vi "_main__.vi"() -> ()   [LabVIEW 2015]
doc: "PKT-8 based Magnitometer"
uses:
  <vilib>/NI/Modbus Library/API/Master/Modbus Master.lvclass
  Load and Save Controls_LV2009.llb/RWC_Actions.ctl
  <vilib>/Utility/error.llb/DialogType.ctl
panel:
  out "ch8_z":dbl format="%.1f"
  out "ch7_z":dbl format="%.1f"
  out "ch6_z":dbl format="%.1f"
  out "ch5_z":dbl format="%.1f"
  out "ch4_z":dbl format="%.1f"
  out "ch3_z":dbl format="%.1f"
  out "ch2_z":dbl format="%.1f"
  out "ch1_z":dbl format="%.1f"
  out "new point":bool=TRUE
  out "статус":bool
  in  "счетчик":u16
  in  "Tab Control":enum32{"Изм.", "Н 1", "Н 2"}(tab)
  in  "show graph B":bool
  in  "show graph U":bool
  out "U8":dbl format="%.1f"
  out "U7":dbl format="%.1f"
  out "U6":dbl format="%.1f"
  out "U5":dbl format="%.1f"
  out "U4":dbl format="%.1f"
  out "U3":dbl format="%.1f"
  out "U2":dbl format="%.1f"
  out "U1":dbl format="%.1f"
  out "8":dbl format="%.2f"
  out "7":dbl format="%.2f"
  out "6":dbl format="%.2f"
  out "5":dbl format="%.2f"
  out "4":dbl format="%.2f"
  out "3":dbl format="%.2f"
  out "2":dbl format="%.2f"
  out "1":dbl format="%.3f"
  in  "Режим работы графика":enum32{"Самописец", "Ручное упр."}(radio)
  in  "Add point":bool
  in  "buf en":bool=TRUE caption="1_ch_abs 2"
  in  "buffer":u16=20 min=1 max=128
  in  "SPS":enum16{"2,5 SPS", "5 SPS", "10 SPS"}(ring)=enum."5 SPS"
  in  "ID":u8=102
  in  "Порт":u16
  in  "IP":string
  in  "Пароль":string
  out "refnum out":refnum<file>
  in  "stop":bool
  in  "range":T1(ring)=enum."± 312.5 мВ"
  in  "Set_zero_8":bool
  in  "Set_zero_7":bool
  in  "Set_zero_6":bool
  in  "Set_zero_5":bool
  in  "Set_zero_4":bool
  in  "Set_zero_3":bool
  in  "Set_zero_2":bool
  in  "Set_zero_1":bool
  in  "канал 1":dbl=76.0 format="%#_4g"
  in  "канал 2":dbl=76.0 format="%#_4g"
  in  "канал 3":dbl=76.0 format="%#_4g"
  in  "канал 4":dbl=76.0 format="%#_4g"
  in  "канал 5":dbl=76.0 format="%#_4g"
  in  "канал 6":dbl=76.0 format="%#_4g"
  in  "канал 7":dbl=76.0 format="%#_4g"
  in  "канал 8":dbl=76.0 format="%#_4g"
  in  "Сохранение в файл":bool=TRUE
  in  "интервал, сек.":u16=30 min=1 max=3600 step=1
  out "Path":string
  out "File header exist?":bool caption="Disconn"
  out "Соед.":refnum<class "Modbus Master.lvclass">
  # "№"
  # "B [ mT ]"
  # "U [ uV ]"
  # "Настройки АЦП"
  # "Буфер. усреднения"
  # "Скорость измерений"
  # "SPS = Samples Per Sec."
  # "Диапазон"
  # "Входной буфер АЦП"
  # "Настройки соединения"
  # "Пароль"
  # "Коэффициенты, uV/mT"
  # "Установка нуля"
  # "Настройки сохранения"
types:
  T1 = enum16{"", "± 2.5 В", "± 1.25 В", "± 0.625 В", "± 312.5 мВ", "± 156.25 мВ", "± 78.125 мВ"}
  T2 = typedef "DialogType.ctl" = u16
  T3 = typedef "RWC_Actions.ctl" = enum16{"Read", "Write", "Read and Create"}
  T4 = enum8{"Enabled", "Disabled", "Disabled and Grayed Out"}
  T5 = cluster{"U1":dbl, "U2":dbl, "U3":dbl, "U4":dbl, "U5":dbl, "U6":dbl, "U7":dbl, "U8":dbl}
  T6 = cluster{"1":dbl, "2":dbl, "3":dbl, "4":dbl, "5":dbl, "6":dbl, "7":dbl, "8":dbl}
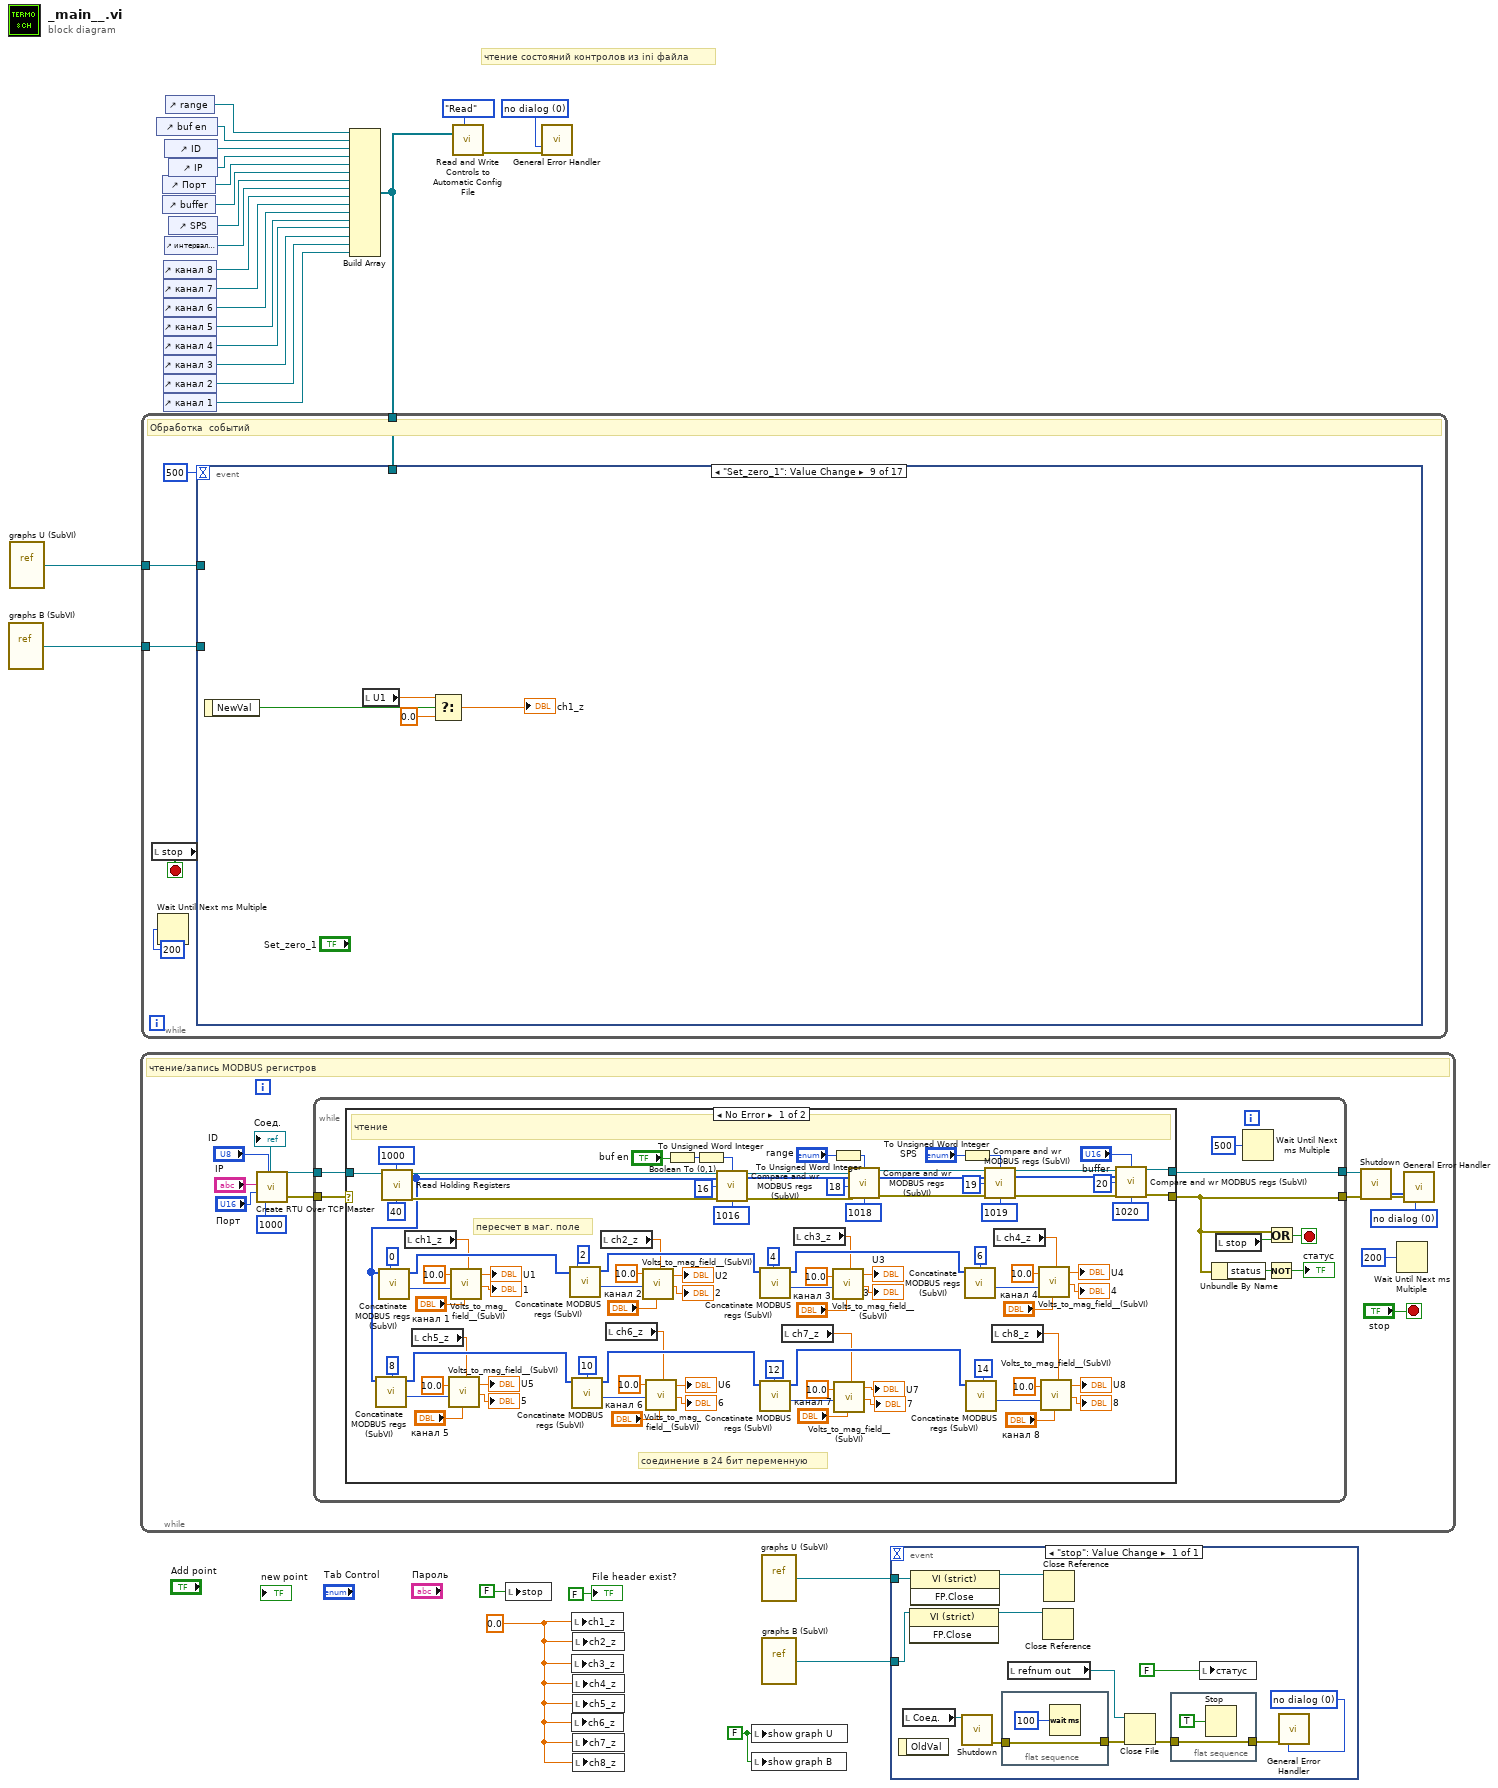
[diagram p0: block diagram]
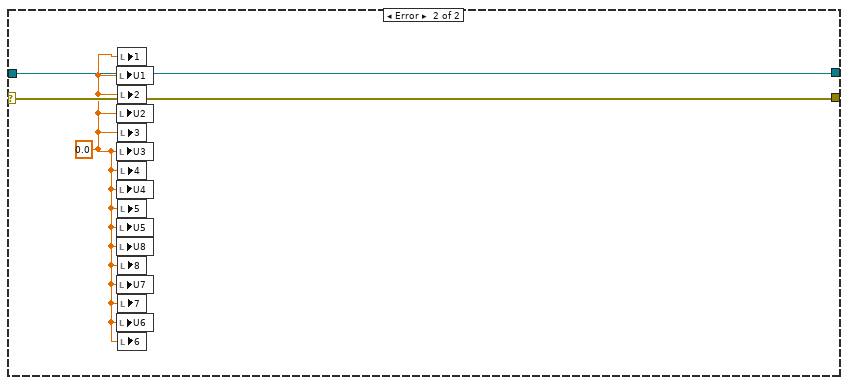
[diagram p2: hidden frame]
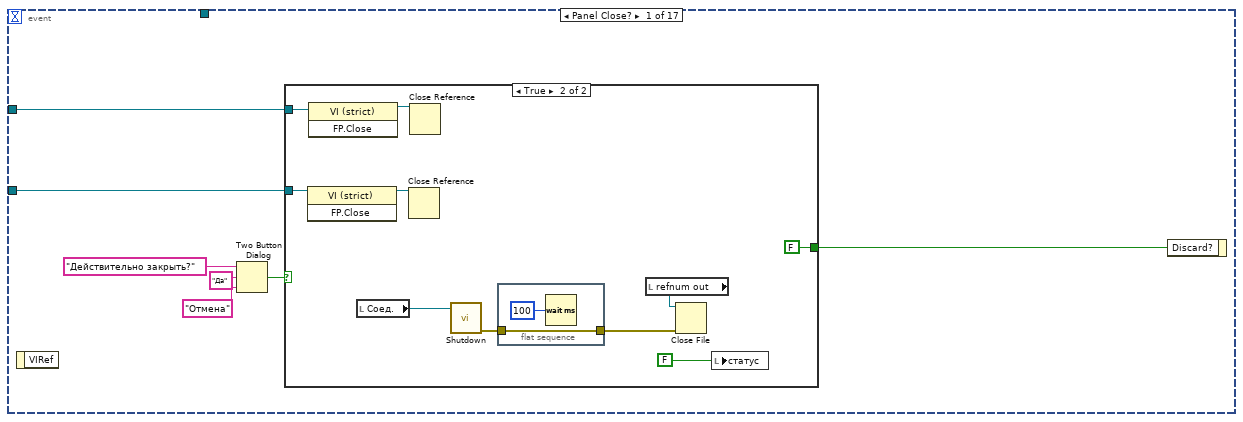
[diagram p3: hidden frame]
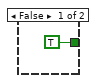
[diagram p4: hidden frame]
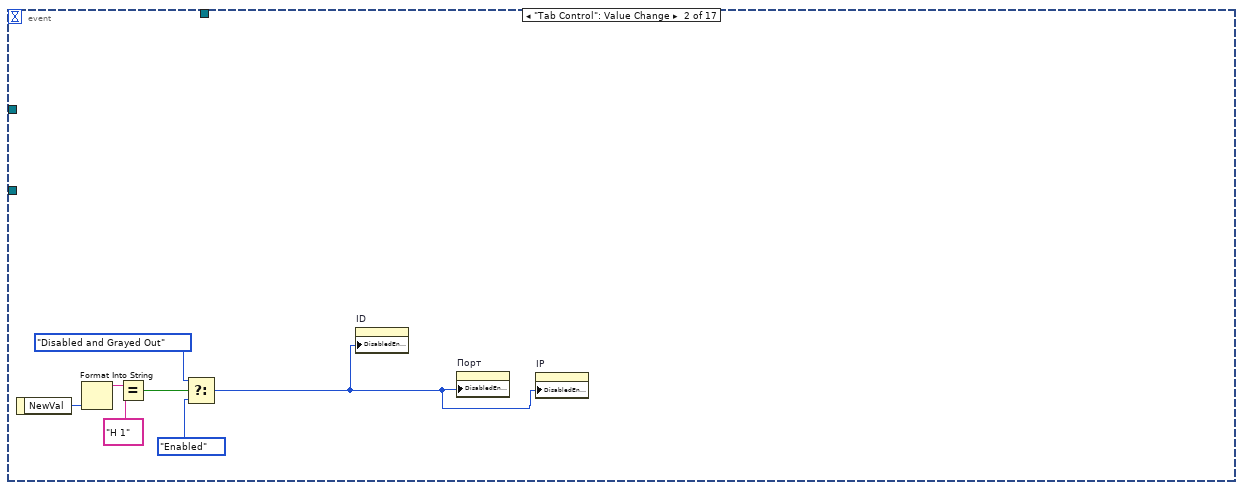
[diagram p5: hidden frame]
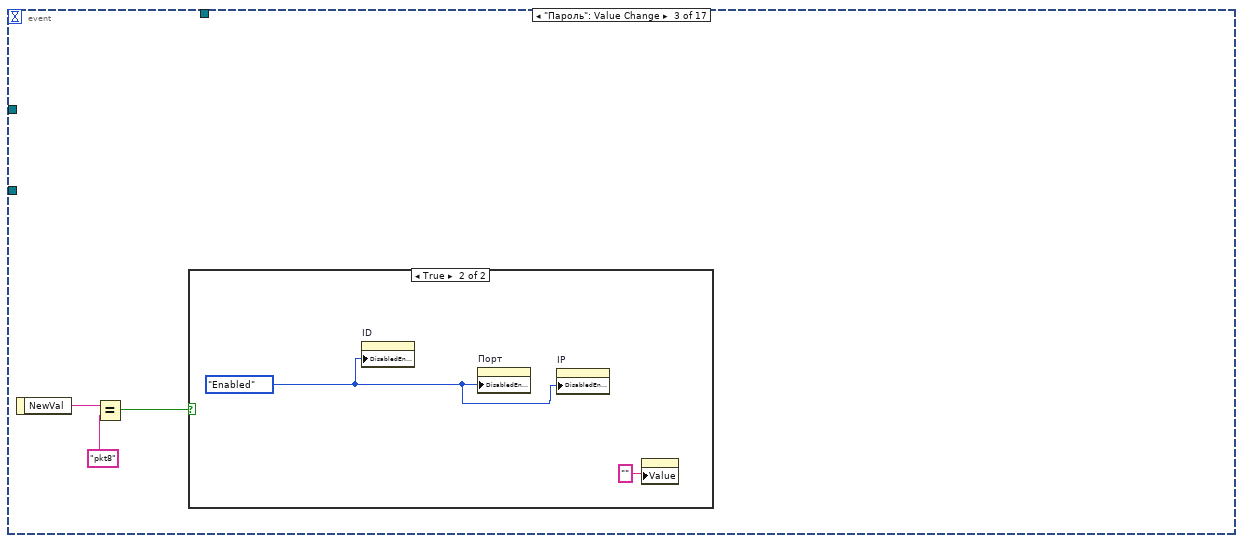
[diagram p6: hidden frame]
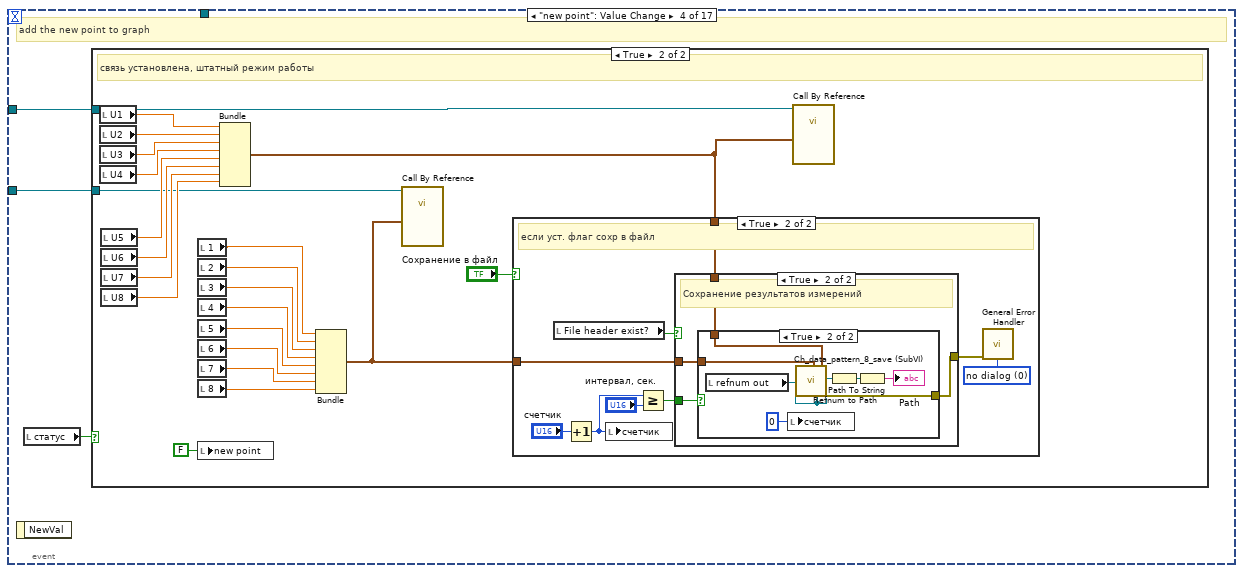
[diagram p8: hidden frame]
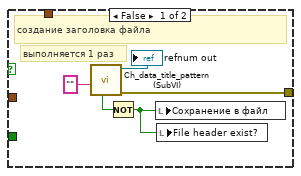
[diagram p11: hidden frame]
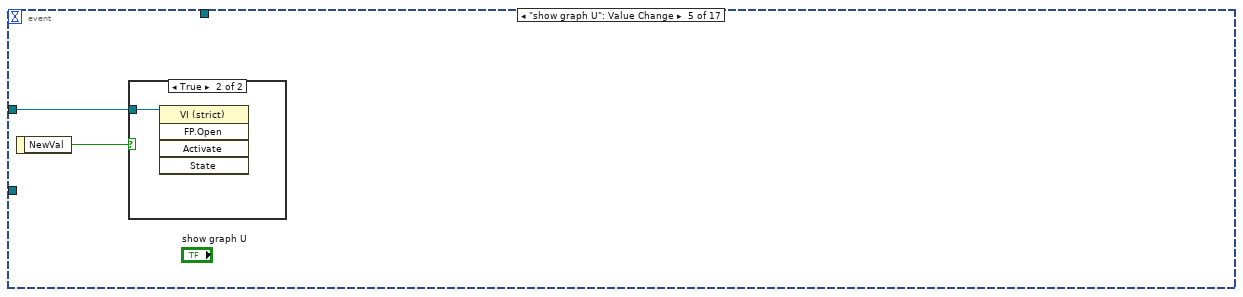
[diagram p13: hidden frame]
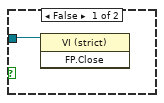
[diagram p14: hidden frame]
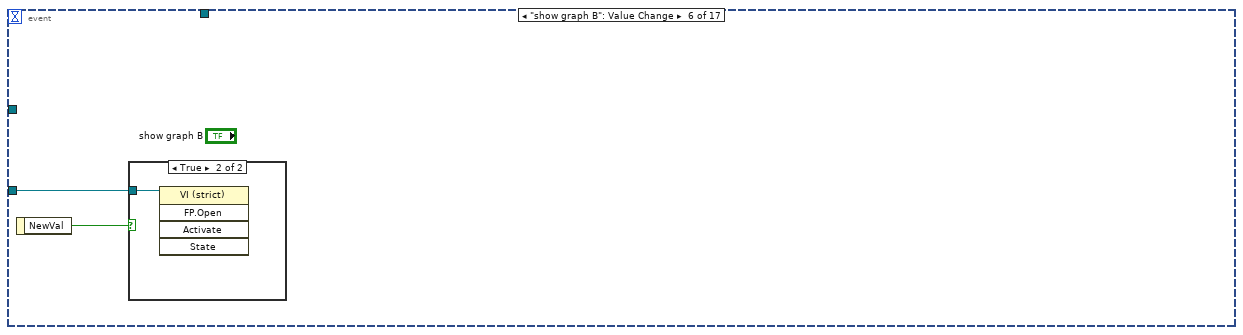
[diagram p15: hidden frame]
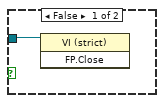
[diagram p16: hidden frame]
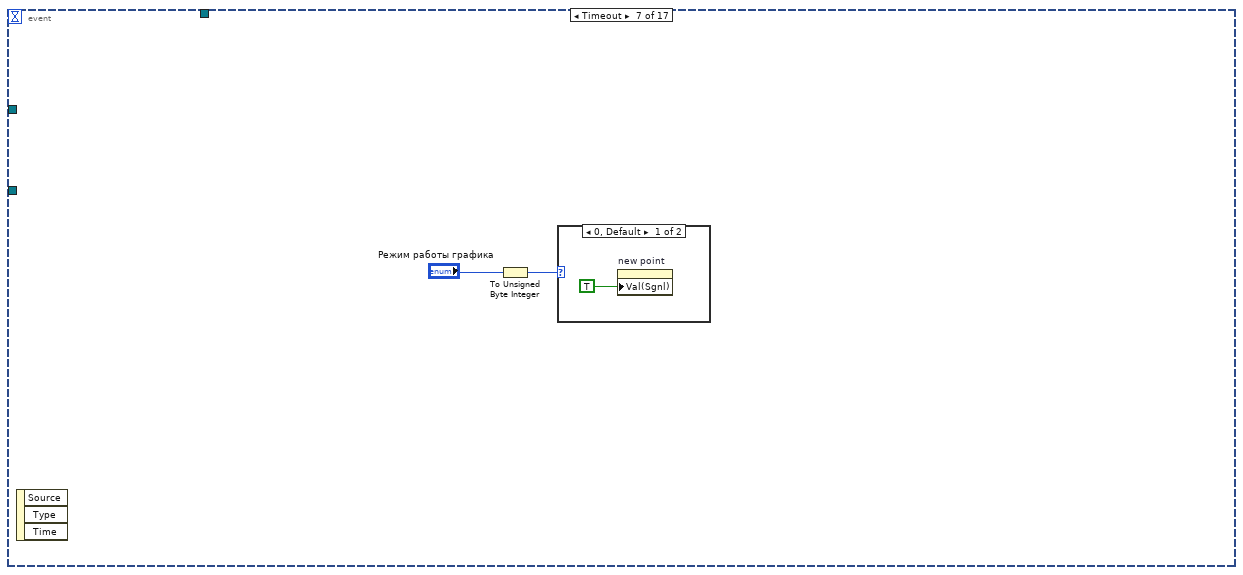
[diagram p17: hidden frame]
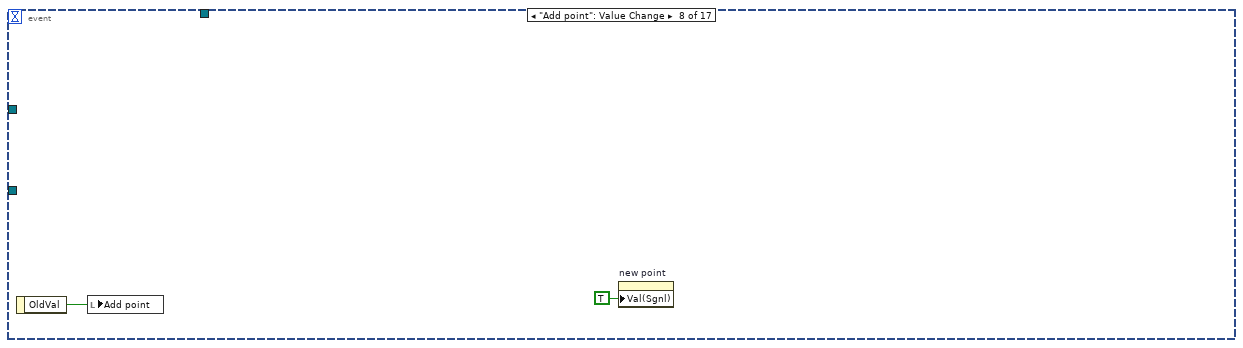
[diagram p19: hidden frame]
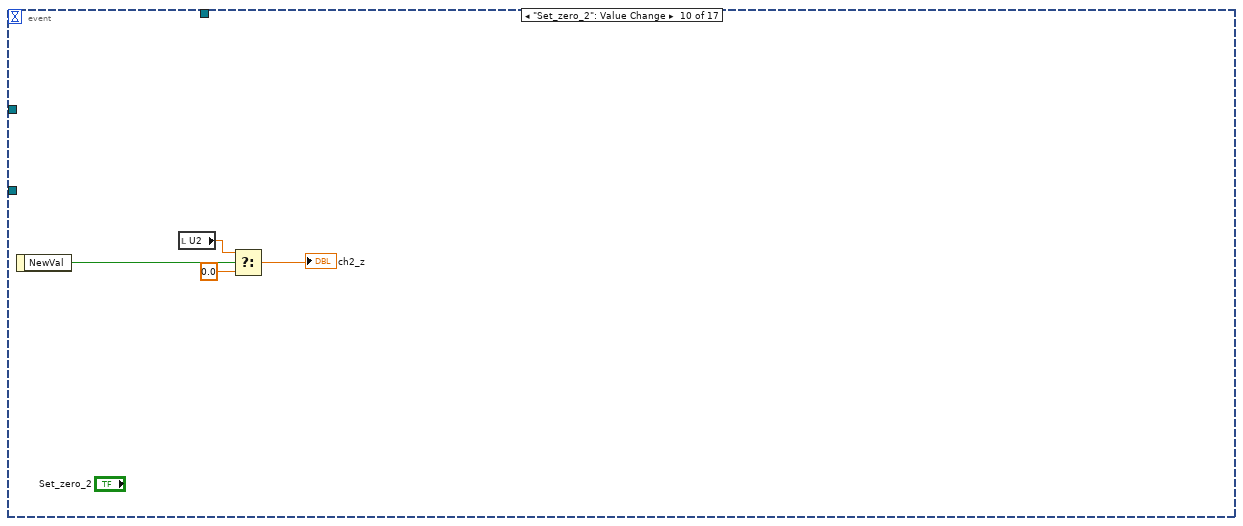
[diagram p20: hidden frame]
diagram:
  w2 = 0.0 ("U1")
  w4 = FALSE ("show graph U")
  w20 = T2 0 items=["no dialog", "OK message", "continue or stop message", "OK message + warnings", "continue/stop + warnings"] ("type of dialog (OK msg:1)")
  # "чтение состояний контролов из ini файла"
  n1 = vi-ref "graphs B (SubVI).vi"() -> (w5:refnum<vi>)
  n2 = vi-ref "graphs U (SubVI).vi"() -> (w8:refnum<vi>)
  n3 = while {
    stop <- "stop" stop-if-true
    w32 = T2 0 items=["no dialog", "OK message", "continue or stop message", "OK message + warnings", "continue/stop + warnings"] ("type of dialog (OK msg:1)")
    # "чтение/запись MODBUS регистров"
    n4 = call "Create RTU Over TCP Master.vi"("unit ID"="ID", "connect timeout ms"=1000, "port (502)"="Порт", "address"="IP") -> ("error out"=w36:errorcluster, "TCP master instance"=w37:refnum<class "Modbus Master.lvclass">)  [unwired: 6 in]
    "Соед." <- w37
    n5 = while {
      tunnel: w37 -> [w49]
      tunnel: w36 -> [w48]
      tunnel: [w42] -> w35
      tunnel: [w47] -> w34
      stop <- w45 stop-if-true
      n6 = case shown="No Error" w48 {
        selector: w48 -> [_ w146]
        tunnel: w49 -> [w142 w147]
        tunnel: [w99 w146] -> w42
        tunnel: [w100 w147] -> w47
        frame No Error {
          # "пересчет в маг. поле"
          # "соединение в 24 бит переменную"
          # "чтение"
          n7 = call-dynamic "Read Holding Registers.vi"("number of inputs"=u16 40, "starting address"=u16 1000, "Modbus master in"=w142) -> ("error out"=w101:errorcluster, "register values"=w58:u16[], "Modbus master out"=w102:refnum<class "Modbus Master.lvclass">)  [unwired: 6 in]
          n8 = call "Concatinate MODBUS regs (SubVI).vi"("LSB reg num"=u16 8, "registers array in"=w58) -> ("register data"=w124:i32, "registers array out"=w86:u16[])  [unwired: 8 in]
          n9 = call "Concatinate MODBUS regs (SubVI).vi"("LSB reg num"=u16 0, "registers array in"=w58) -> ("register data"=w129:i32, "registers array out"=w89:u16[])  [unwired: 8 in]
          n10 = local read "ch1_z"() -> (w57:dbl)
          n11 = local read "ch5_z"() -> (w53:dbl)
          n12 = call "Volts_to_mag_field__(SubVI).vi"("делитель"=10.0, "U"=w124, "k"="канал 5", "zero lvl"=w53) -> ("meas_voltage"=→"U5":dbl, "B"=→"5":dbl)  [unwired: 20 in, 2 out]
          n13 = call "Volts_to_mag_field__(SubVI).vi"("делитель"=10.0, "U"=w129, "k"="канал 1", "zero lvl"=w57) -> ("meas_voltage"=→"U1":dbl, "B"=→"1":dbl)  [unwired: 20 in, 2 out]
          n14 = call "Concatinate MODBUS regs (SubVI).vi"("LSB reg num"=u16 2, "registers array in"=w89) -> ("register data"=w128:i32, "registers array out"=w88:u16[])  [unwired: 8 in]
          n15 = call "Concatinate MODBUS regs (SubVI).vi"("LSB reg num"=u16 10, "registers array in"=w86) -> ("register data"=w123:i32, "registers array out"=w85:u16[])  [unwired: 8 in]
          n16 = local read "ch2_z"() -> (w56:dbl)
          n17 = local read "ch6_z"() -> (w52:dbl)
          n18 = call "Volts_to_mag_field__(SubVI).vi"("делитель"=10.0, "U"=w128, "k"="канал 2", "zero lvl"=w56) -> ("meas_voltage"=→"U2":dbl, "B"=→"2":dbl)  [unwired: 20 in, 2 out]
          n19 = call "Volts_to_mag_field__(SubVI).vi"("делитель"=10.0, "U"=w123, "k"="канал 6", "zero lvl"=w52) -> ("meas_voltage"=→"U6":dbl, "B"=→"6":dbl)  [unwired: 20 in, 2 out]
          n20 = Boolean To (0,1)(Boolean="buf en") -> (0, 1=w71:i16)
          n21 = To Unsigned Word Integer(number=w71) -> (unsigned 16bit integer=w70:u16)
          n22 = call "Compare and wr MODBUS regs (SubVI).vi"("Modbus Master in"=w102, "control"=w70, "modbus read arr in"=w58, "arr el. index"=16 ("arr element"), "error in (no error)"=w101, "reg address"=u16 1016 ("starting address")) -> ("Modbus Master out"=w81:refnum<class "Modbus Master.lvclass">, "modbus read arr  out"=w83:u16[], "error out"=w82:errorcluster)  [unwired: 7 in]
          n23 = call "Concatinate MODBUS regs (SubVI).vi"("LSB reg num"=u16 4, "registers array in"=w88) -> ("register data"=w127:i32, "registers array out"=w87:u16[])  [unwired: 8 in]
          n24 = call "Concatinate MODBUS regs (SubVI).vi"("LSB reg num"=u16 12, "registers array in"=w85) -> ("register data"=w122:i32, "registers array out"=w84:u16[])  [unwired: 8 in]
          n25 = local read "ch7_z"() -> (w51:dbl)
          n26 = local read "ch3_z"() -> (w55:dbl)
          n27 = To Unsigned Word Integer(number="range") -> (unsigned 16bit integer=w67:u16)
          n28 = call "Volts_to_mag_field__(SubVI).vi"("делитель"=10.0, "U"=w127, "k"="канал 3", "zero lvl"=w55) -> ("meas_voltage"=→"U3":dbl, "B"=→"3":dbl)  [unwired: 20 in, 2 out]
          n29 = call "Volts_to_mag_field__(SubVI).vi"("делитель"=10.0, "U"=w122, "k"="канал 7", "zero lvl"=w51) -> ("meas_voltage"=→"U7":dbl, "B"=→"7":dbl)  [unwired: 20 in, 2 out]
          n30 = call "Compare and wr MODBUS regs (SubVI).vi"("Modbus Master in"=w81, "control"=w67, "modbus read arr in"=w83, "arr el. index"=18 ("arr element"), "error in (no error)"=w82, "reg address"=u16 1018 ("starting address")) -> ("Modbus Master out"=w79:refnum<class "Modbus Master.lvclass">, "modbus read arr  out"=w78:u16[], "error out"=w80:errorcluster)  [unwired: 7 in]
          n31 = To Unsigned Word Integer(number="SPS") -> (unsigned 16bit integer=w63:u16)
          n32 = call "Concatinate MODBUS regs (SubVI).vi"("LSB reg num"=u16 6, "registers array in"=w87) -> ("register data"=w125:i32)  [unwired: 8 in, 1 out]
          n33 = call "Concatinate MODBUS regs (SubVI).vi"("LSB reg num"=u16 14, "registers array in"=w84) -> ("register data"=w121:i32)  [unwired: 8 in, 1 out]
          n34 = call "Compare and wr MODBUS regs (SubVI).vi"("Modbus Master in"=w79, "control"=w63, "modbus read arr in"=w78, "arr el. index"=19 ("arr element"), "error in (no error)"=w80, "reg address"=u16 1019 ("starting address")) -> ("Modbus Master out"=w76:refnum<class "Modbus Master.lvclass">, "modbus read arr  out"=w75:u16[], "error out"=w77:errorcluster)  [unwired: 7 in]
          n35 = local read "ch8_z"() -> (w50:dbl)
          n36 = local read "ch4_z"() -> (w54:dbl)
          n37 = call "Volts_to_mag_field__(SubVI).vi"("делитель"=10.0, "U"=w125, "k"="канал 4", "zero lvl"=w54) -> ("meas_voltage"=→"U4":dbl, "B"=→"4":dbl)  [unwired: 20 in, 2 out]
          n38 = call "Volts_to_mag_field__(SubVI).vi"("делитель"=10.0, "U"=w121, "k"="канал 8", "zero lvl"=w50) -> ("meas_voltage"=→"U8":dbl, "B"=→"8":dbl)  [unwired: 20 in, 2 out]
          n39 = call "Compare and wr MODBUS regs (SubVI).vi"("Modbus Master in"=w76, "control"="buffer", "modbus read arr in"=w75, "arr el. index"=20 ("arr element"), "error in (no error)"=w77, "reg address"=u16 1020 ("starting address")) -> ("Modbus Master out"=w100:refnum<class "Modbus Master.lvclass">, "error out"=w99:errorcluster)  [unwired: 7 in, 1 out]
        }
        frame Error {
          w145 = 0.0 ("T1")
          n40 = local write "U1"(w145) -> ()
          n41 = local write "U2"(w145) -> ()
          n42 = local write "U3"(w145) -> ()
          n43 = local write "U4"(w145) -> ()
          n44 = local write "U5"(w145) -> ()
          n45 = local write "U8"(w145) -> ()
          n46 = local write "U7"(w145) -> ()
          n47 = local write "U6"(w145) -> ()
          n48 = local write "1"(w145) -> ()
          n49 = local write "2"(w145) -> ()
          n50 = local write "3"(w145) -> ()
          n51 = local write "4"(w145) -> ()
          n52 = local write "5"(w145) -> ()
          n53 = local write "8"(w145) -> ()
          n54 = local write "7"(w145) -> ()
          n55 = local write "6"(w145) -> ()
        }
      }
      n56 = Unbundle By Name(w42) -> ("status"=w44:bool)
      n57 = local read "stop"() -> (w46:bool)
      n58 = Wait Until Next ms Multiple(millisecond multiple=u32 500) -> ()  [unwired: 1 out]
      n59 = Not(x=w44) -> (.not. x?=→"статус":bool)
      n60 = Or(x=w42, y=w46) -> (x .or. y?=w45:bool)
    }
    n61 = call-dynamic "Shutdown.vi"("error in"=w35, "Modbus master in"=w34) -> ("error out"=w33:errorcluster)  [unwired: 9 in]
    n62 = Wait Until Next ms Multiple(millisecond multiple=u32 200) -> ()  [unwired: 1 out]
    n63 = call <vilib>:"General Error Handler.vi"("type of dialog (OK msg:1)"=w32, "error in (no error)"=w33) -> ()  [unwired: 1 in, 13 out]
  }
  n64 = control-ref of="buf en"() -> (w6:refnum<vi>)
  n65 = control-ref of="Порт"() -> (w18:refnum<vi>)
  n66 = control-ref of="buffer"() -> (w17:refnum<vi>)
  n67 = control-ref of="канал 8"() -> (w16:refnum<vi>)
  n68 = control-ref of="канал 7"() -> (w15:refnum<vi>)
  n69 = control-ref of="канал 6"() -> (w14:refnum<vi>)
  n70 = control-ref of="канал 5"() -> (w13:refnum<vi>)
  n71 = control-ref of="канал 4"() -> (w12:refnum<vi>)
  n72 = control-ref of="канал 3"() -> (w11:refnum<vi>)
  n73 = control-ref of="канал 2"() -> (w10:refnum<vi>)
  n74 = control-ref of="канал 1"() -> (w9:refnum<vi>)
  n75 = control-ref of="ID"() -> (w26:refnum<vi>)
  n76 = control-ref of="интервал, сек."() -> (w23:refnum<vi>)
  n77 = control-ref of="range"() -> (w1:refnum<vi>)
  n78 = control-ref of="IP"() -> (w25:refnum<vi>)
  n79 = control-ref of="SPS"() -> (w24:refnum<vi>)
  n80 = Build Array(w1, w6, w26, w25, w18, w17, w24, w23, w16, w15, w14, w13, w12, w11, w10, w9) -> (w19:refnum<vi>[])
  n81 = while {
    tunnel: w19 -> [w151]
    tunnel: w8 -> [w149]
    tunnel: w5 -> [w148]
    stop <- w152 stop-if-true
    # "Обработка  событий"
    n82 = local read "stop"() -> (w152:bool)
    n83 = Wait Until Next ms Multiple(millisecond multiple=u32 200) -> ()  [unwired: 1 out]
    n84 = event shown="[8] \"Set_zero_1\": Value Change" {
      selector: _ -> [_ _ _ _ _ _ _ _ _ _ _ _ _ _ _ _ _]
      dyn-events: _ -> [_ _ _ _ _ _ _ _ _ _ _ _ _ _ _ _ _]
      timeout: 500 -> [_ _ _ _ _ _ _ _ _ _ _ _ _ _ _ _ _]
      tunnel: w151 -> [_ _ _ _ _ _ _ _ _ _ _ _ _ _ _ _ w284]
      tunnel: w149 -> [w155 _ _ w187 w237 _ _ _ _ _ _ _ _ _ _ _ _]
      tunnel: w148 -> [w154 _ _ w186 _ w240 _ _ _ _ _ _ _ _ _ _ _]
      event Panel Close? {
        n85 = event-data() -> ()  [unwired: 2 out]
        n86 = Two Button Dialog(message="Действительно закрыть?", 1:"Отмена" ("T button name (\"OK\")"), 2:"Да" ("T button name (\"OK\")")) -> (T button?=w160:bool)
        n87 = case shown="True" w160 {
          tunnel: [TRUE ("Discard?") FALSE ("Discard?")] -> w156
          tunnel: w155 -> [_ w165]
          tunnel: w154 -> [_ w162]
          frame False {
          }
          frame True {
            n88 = invoke class="VI (strict)" method="FP.Close"(reference=w162) -> (reference out=w163:refnum<vi>)  [unwired: 2 in, 2 out]
            n89 = invoke class="VI (strict)" method="FP.Close"(reference=w165) -> (reference out=w164:refnum<vi>)  [unwired: 2 in, 2 out]
            n90 = local read "Соед."() -> (w170:refnum<class "Modbus Master.lvclass">)
            n91 = Close Reference(reference=w163) -> ()  [unwired: 1 in, 1 out]
            n92 = Close Reference(reference=w164) -> ()  [unwired: 1 in, 1 out]
            n93 = call-dynamic "Shutdown.vi"("Modbus master in"=w170) -> ("error out"=w169:errorcluster)  [unwired: 10 in]
            n94 = flat-sequence {
              tunnel: w169 -> [w172]
              tunnel: [w172] -> w168
              frame #0 {
                n95 = Wait (ms)(milliseconds to wait=u32 100) -> ()  [unwired: 1 out]
              }
            }
            n96 = local read "refnum out"() -> (w166:refnum<file>)
            n97 = Close File(refnum=w166, error in=w168) -> ()  [unwired: 2 out]
            n98 = local write "статус"(FALSE ("Связь с блоком 4")) -> ()
          }
        }
        n99 = event-data("Discard?"=w156) -> ()  [unwired: 1 in, 1 out]
      }
      event "Tab Control": Value Change {
        n100 = event-data() -> ("NewVal"=w180:enum32{"Изм.", "Н 1", "Н 2"})  [unwired: 1 out]
        n101 = Format Into String(w180) -> (resulting string=w179:string)  [unwired: 3 in, 1 out]
        n102 = Equal?(x=w179, y="Н 1") -> (x = y?=w177:bool)
        n103 = Select(t=T4."Disabled and Grayed Out" ("Disabled"), s=w177, f=T4."Enabled" ("Disabled")) -> (s? t:f=w174:T4)
        n104 = property on="ID" class="DigNum (strict)"("DisabledEnum"=w174) -> ()  [unwired: 2 in, 2 out]
        n105 = property on="Порт" class="DigNum (strict)"("DisabledEnum"=w174) -> ()  [unwired: 2 in, 2 out]
        n106 = property on="IP" class="Str"("DisabledEnum"=w174) -> ()  [unwired: 2 in, 2 out]
      }
      event "Пароль": Value Change {
        n107 = event-data() -> ("NewVal"=w182:string)  [unwired: 1 out]
        n108 = Equal?(x=w182, y="pkt8") -> (x = y?=w181:bool)
        n109 = case shown="True" w181 {
          frame False {
          }
          frame True {
            w184 = T4."Enabled" ("Disabled")
            n110 = property on="ID" class="DigNum (strict)"("DisabledEnum"=w184) -> ()  [unwired: 2 in, 2 out]
            n111 = property on="Порт" class="DigNum (strict)"("DisabledEnum"=w184) -> ()  [unwired: 2 in, 2 out]
            n112 = property on="IP" class="Str"("DisabledEnum"=w184) -> ()  [unwired: 2 in, 2 out]
            n113 = property on="Пароль" class="Str"("Value"="" ("Пароль")) -> ()  [unwired: 2 in, 2 out]
          }
        }
      }
      event "new point": Value Change {
        # "add the new point to graph"
        n114 = event-data() -> ()  [unwired: 2 out]
        n115 = local read "статус"() -> (w188:bool)
        n116 = case shown="True" w188 {
          tunnel: w187 -> [_ w192]
          tunnel: w186 -> [_ w190]
          frame False {
            # "нет связи"
          }
          frame True {
            # "связь установлена, штатный режим работы"
            n117 = local read "U1"() -> (w201:dbl)
            n118 = local read "U2"() -> (w210:dbl)
            n119 = local read "U3"() -> (w209:dbl)
            n120 = local read "U4"() -> (w208:dbl)
            n121 = local read "U5"() -> (w204:dbl)
            n122 = local read "U6"() -> (w205:dbl)
            n123 = local read "U7"() -> (w206:dbl)
            n124 = local read "U8"() -> (w207:dbl)
            n125 = local read "1"() -> (w200:dbl)
            n126 = local read "2"() -> (w199:dbl)
            n127 = local read "3"() -> (w198:dbl)
            n128 = local read "4"() -> (w197:dbl)
            n129 = local read "5"() -> (w196:dbl)
            n130 = local read "6"() -> (w195:dbl)
            n131 = local read "7"() -> (w194:dbl)
            n132 = local read "8"() -> (w193:dbl)
            n133 = local write "new point"(FALSE ("new point")) -> ()
            n134 = Bundle("U1"=w201, "U2"=w210, "U3"=w209, "U4"=w208, "U5"=w204, "U6"=w205, "U7"=w206, "U8"=w207) -> (w191:T5)  [unwired: 1 in]
            n135 = Bundle("1"=w200, "2"=w199, "3"=w198, "4"=w197, "5"=w196, "6"=w195, "7"=w194, "8"=w193) -> (w189:T6)  [unwired: 1 in]
            n136 = call-by-ref "Call By Reference"(reference=w190, "Cluster"=w189) -> ()  [unwired: 12 in, 2 out]
            n137 = case shown="True" "Сохранение в файл" {
              tunnel: w191 -> [_ w212]
              tunnel: w189 -> [_ w211]
              frame False {
              }
              frame True {
                w219 = T2 0 items=["no dialog", "OK message", "continue or stop message", "OK message + warnings", "continue/stop + warnings"] ("type of dialog (OK msg:1)")
                # "если уст. флаг сохр в файл"
                n138 = local read "File header exist?"() -> (w214:bool)
                n139 = Increment(x="счетчик") -> (x+1=w216:u16)
                n140 = local write "счетчик"(w216) -> ()
                n141 = Greater Or Equal?(x=w216, y="интервал, сек.") -> (x >= y?=w215:bool)
                n142 = case shown="True" w214 {
                  tunnel: [w222 w227] -> w218
                  tunnel: w215 -> [_ w228]
                  tunnel: w212 -> [_ w226]
                  tunnel: w211 -> [_ w225]
                  frame False {
                    # "выполняется 1 раз"
                    # "создание заголовка файла"
                    n143 = call "Ch_data_title_pattern (SubVI).vi"("Единица измерений"="") -> ("error out"=w222:errorcluster, "Byte Stream File out"=→"refnum out":refnum<file>, "cancelled"=w221:bool)  [unwired: 7 in, 1 out]
                    n144 = Not(x=w221) -> (.not. x?=w220:bool)
                    n145 = local write "Сохранение в файл"(w220) -> ()
                    n146 = local write "File header exist?"(w220) -> ()
                  }
                  frame True {
                    # "Сохранение результатов измерений"
                    n147 = case shown="True" w228 {
                      tunnel: [_ w232] -> w227
                      tunnel: w226 -> [_ w231]
                      tunnel: w225 -> [_ w230]
                      frame False {
                      }
                      frame True {
                        n148 = local read "refnum out"() -> (w229:refnum<file>)
                        n149 = local write "счетчик"(u8 0 ("счетчик")) -> ()
                        n150 = call "Ch_data_pattern_8_save (SubVI).vi"("B Cluster"=w230, "file"=w229, "U cluster"=w231) -> ("error out"=w232:errorcluster)  [unwired: 24 in]
                        n151 = Refnum to Path(1:w229) -> (0:w235:path)
                        n152 = Path To String(path=w235) -> (string=→"Path":string)
                      }
                    }
                  }
                }
                n153 = call <vilib>:"General Error Handler.vi"("type of dialog (OK msg:1)"=w219, "error in (no error)"=w218) -> ()  [unwired: 1 in, 13 out]
              }
            }
            n154 = call-by-ref "Call By Reference"(reference=w192, "Cluster"=w191) -> ()  [unwired: 12 in, 2 out]
          }
        }
      }
      event "show graph U": Value Change {
        n155 = event-data() -> ("NewVal"=w236:bool)  [unwired: 1 out]
        n156 = case shown="True" w236 {
          tunnel: w237 -> [w238 w239]
          frame False {
            n157 = invoke class="VI (strict)" method="FP.Close"(reference=w238) -> ()  [unwired: 2 in, 3 out]
          }
          frame True {
            n158 = invoke class="VI (strict)" method="FP.Open"(reference=w239) -> ()  [unwired: 4 in, 5 out]
          }
        }
      }
      event "show graph B": Value Change {
        n159 = event-data() -> ("NewVal"=w241:bool)  [unwired: 1 out]
        n160 = case shown="True" w241 {
          tunnel: w240 -> [w242 w243]
          frame False {
            n161 = invoke class="VI (strict)" method="FP.Close"(reference=w242) -> ()  [unwired: 2 in, 3 out]
          }
          frame True {
            n162 = invoke class="VI (strict)" method="FP.Open"(reference=w243) -> ()  [unwired: 4 in, 5 out]
          }
        }
      }
      event Timeout {
        n163 = event-data() -> ()  [unwired: 4 out]
        n164 = To Unsigned Byte Integer(number="Режим работы графика") -> (unsigned 8bit integer=w244:u8)
        n165 = case shown="0, Default" w244 {
          frame 0, Default {
            n166 = property on="new point" class="Bool (strict)"("Val(Sgnl)"=TRUE ("add point")) -> ()  [unwired: 2 in, 2 out]
          }
          frame 1 {
          }
        }
      }
      event "Add point": Value Change {
        n167 = event-data() -> ("OldVal"=w247:bool)  [unwired: 1 out]
        n168 = local write "Add point"(w247) -> ()
        n169 = property on="new point" class="Bool (strict)"("Val(Sgnl)"=TRUE ("Value (Signaling)")) -> ()  [unwired: 2 in, 2 out]
      }
      event "Set_zero_1": Value Change {
        n170 = event-data() -> ("NewVal"=w252:bool)  [unwired: 1 out]
        n171 = local read "U1"() -> (w251:dbl)
        n172 = Select(t=w251, s=w252, f=0.0) -> (s? t:f=→"ch1_z":dbl)
      }
      event "Set_zero_2": Value Change {
        n173 = event-data() -> ("NewVal"=w255:bool)  [unwired: 1 out]
        n174 = local read "U2"() -> (w254:dbl)
        n175 = Select(t=w254, s=w255, f=0.0) -> (s? t:f=→"ch2_z":dbl)
      }
      event "Set_zero_3": Value Change {
        n176 = event-data() -> ("NewVal"=w259:bool)  [unwired: 1 out]
        n177 = local read "U3"() -> (w258:dbl)
        n178 = Select(t=w258, s=w259, f=0.0) -> (s? t:f=→"ch3_z":dbl)
      }
      event "Set_zero_4": Value Change {
        n179 = event-data() -> ("NewVal"=w263:bool)  [unwired: 1 out]
        n180 = local read "U4"() -> (w262:dbl)
        n181 = Select(t=w262, s=w263, f=0.0) -> (s? t:f=→"ch4_z":dbl)
      }
      event "Set_zero_5": Value Change {
        n182 = event-data() -> ("NewVal"=w267:bool)  [unwired: 1 out]
        n183 = local read "U5"() -> (w266:dbl)
        n184 = Select(t=w266, s=w267, f=0.0) -> (s? t:f=→"ch5_z":dbl)
      }
      event "Set_zero_6": Value Change {
        n185 = event-data() -> ("NewVal"=w271:bool)  [unwired: 1 out]
        n186 = local read "U6"() -> (w270:dbl)
        n187 = Select(t=w270, s=w271, f=0.0) -> (s? t:f=→"ch6_z":dbl)
      }
      event "Set_zero_7": Value Change {
        n188 = event-data() -> ("NewVal"=w275:bool)  [unwired: 1 out]
        n189 = local read "U7"() -> (w274:dbl)
        n190 = Select(t=w274, s=w275, f=0.0) -> (s? t:f=→"ch7_z":dbl)
      }
      event "Set_zero_8": Value Change {
        n191 = event-data() -> ("NewVal"=w279:bool)  [unwired: 1 out]
        n192 = local read "U8"() -> (w278:dbl)
        n193 = Select(t=w278, s=w279, f=0.0) -> (s? t:f=→"ch8_z":dbl)
      }
      event "IP", "Порт", "buffer", "SPS", "ID", "интервал, сек.", "канал 1", "канал 2", "канал 3", "канал 4", "канал 5", "канал 6", "канал 7", "канал 8", "buf en", "range": Value Change {
        w281 = T2 0 items=["no dialog", "OK message", "continue or stop message", "OK message + warnings", "continue/stop + warnings"] ("type of dialog (OK msg:1)")
        # "запись состояний контролов в ini файл"
        n194 = event-data() -> ()  [unwired: 2 out]
        n195 = call "Read and Write Controls to Automatic Config File.vi"("Action"=RWC_Actions."Write", "Control References"=w284) -> ("error out"=w282:errorcluster)  [unwired: 9 in]
        n196 = call <vilib>:"General Error Handler.vi"("type of dialog (OK msg:1)"=w281, "error in (no error)"=w282) -> ()  [unwired: 1 in, 13 out]
      }
    }
  }
  n197 = call "Read and Write Controls to Automatic Config File.vi"("Action"=RWC_Actions."Read", "Control References"=w19) -> ("error out"=w21:errorcluster)  [unwired: 9 in]
  n198 = local write "stop"(FALSE ("Boolean")) -> ()
  n199 = call <vilib>:"General Error Handler.vi"("type of dialog (OK msg:1)"=w20, "error in (no error)"=w21) -> ()  [unwired: 1 in, 13 out]
  n200 = local write "ch1_z"(w2) -> ()
  n201 = local write "ch3_z"(w2) -> ()
  n202 = local write "ch6_z"(w2) -> ()
  n203 = local write "ch2_z"(w2) -> ()
  n204 = local write "ch4_z"(w2) -> ()
  n205 = local write "ch5_z"(w2) -> ()
  n206 = local write "ch7_z"(w2) -> ()
  n207 = local write "ch8_z"(w2) -> ()
  n208 = local write "show graph U"(w4) -> ()
  n209 = local write "show graph B"(w4) -> ()
  n210 = vi-ref "graphs U (SubVI).vi"() -> (w7:refnum<vi>)
  n211 = vi-ref "graphs B (SubVI).vi"() -> (w3:refnum<vi>)
  n212 = event shown="[0] \"stop\": Value Change" {
    selector: _ -> [_]
    dyn-events: _ -> [_]
    timeout: _ -> [_]
    tunnel: w7 -> [w288]
    tunnel: w3 -> [w286]
    event "stop": Value Change {
      w293 = T2 0 items=["no dialog", "OK message", "continue or stop message", "OK message + warnings", "continue/stop + warnings"] ("type of dialog (OK msg:1)")
      n213 = event-data() -> ()  [unwired: 1 in, 1 out]
      n214 = local read "Соед."() -> (w295:refnum<class "Modbus Master.lvclass">)
      n215 = invoke class="VI (strict)" method="FP.Close"(reference=w286) -> (reference out=w285:refnum<vi>)  [unwired: 2 in, 2 out]
      n216 = invoke class="VI (strict)" method="FP.Close"(reference=w288) -> (reference out=w287:refnum<vi>)  [unwired: 2 in, 2 out]
      n217 = call-dynamic "Shutdown.vi"("Modbus master in"=w295) -> ("error out"=w294:errorcluster)  [unwired: 10 in]
      n218 = flat-sequence {
        tunnel: w294 -> [w299]
        tunnel: [w299] -> w292
        frame #0 {
          n219 = Wait (ms)(milliseconds to wait=u32 100) -> ()  [unwired: 1 out]
        }
      }
      n220 = local read "refnum out"() -> (w296:refnum<file>)
      n221 = Close Reference(reference=w285) -> ()  [unwired: 1 in, 1 out]
      n222 = Close Reference(reference=w287) -> ()  [unwired: 1 in, 1 out]
      n223 = Close File(refnum=w296, error in=w292) -> (error out=w290:errorcluster)  [unwired: 1 out]
      n224 = flat-sequence {
        tunnel: [w297] -> w289
        tunnel: w290 -> [w297]
        frame #0 {
          n225 = Stop(stop? (T)=TRUE) -> ()
        }
      }
      n226 = local write "статус"(FALSE ("Запись в файл")) -> ()
      n227 = call <vilib>:"General Error Handler.vi"("error in (no error)"=w289, "[exception action] (none:0)"=w293) -> ()  [unwired: 2 in, 12 out]
    }
  }
  "File header exist?" <- FALSE ("flag1")
